vi "Find and Highlight Event Frames.vi"(8 "error in":errorcluster, 10 "References":refnum<vi>[](array[refnum]), 11 "Event Name":string) -> (0 "error out":errorcluster)   [LabVIEW 2019, in "Panther Dashboard.lvlib"]
uses:
  Panther Dashboard.lvlib
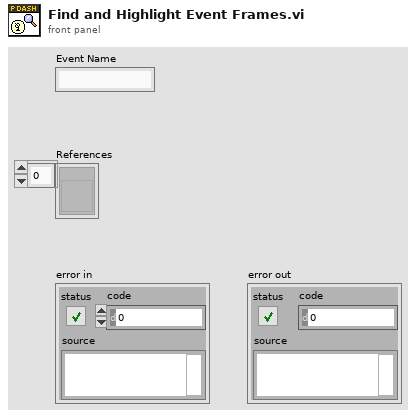
[diagram p1: front panel]
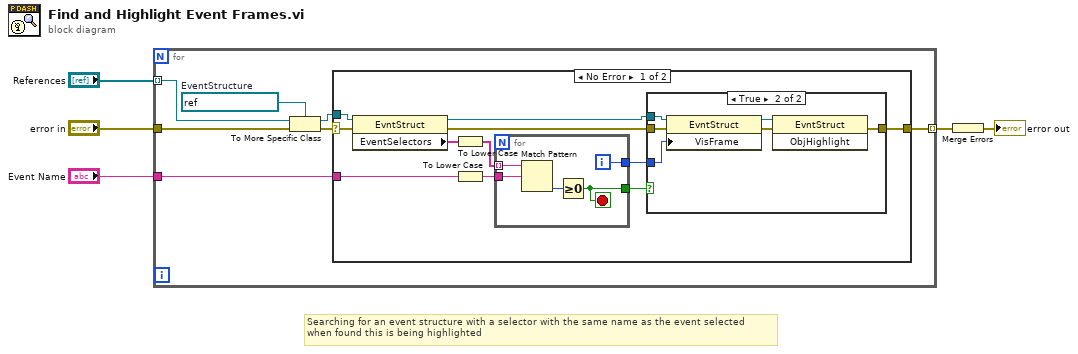
[diagram p0: block diagram]
diagram:
  # "Searching for an event structure with a selector with the same name as the event selected\nwhen found this is being highlighted"
  n1 = for {
    tunnel: "References" -> [w9] mode=indexing
    tunnel: "Event Name" -> [w6]
    tunnel: "error in" -> [w11]
    tunnel: [w10] -> w1 mode=indexing
    w8 = refnum<vi> refnum  # EventStructure
    n2 = To More Specific Class(target class=w8, reference=w9, error in=w11) -> (specific class reference=w7:refnum<vi>, error out=w12:errorcluster)
    n3 = case shown="No Error" w12 {
      selector: w12 -> [w23 _]
      tunnel: w7 -> [w18 _]
      tunnel: w6 -> [w19 _]
      tunnel: [w21 _] -> w10
      frame No Error {
        n4 = property class="EvntStruct"(reference=w18, error in=w23) -> (reference out=w15:refnum<vi>, error out=w22:errorcluster, "EventSelectors"=w20:string[])
        n5 = To Lower Case(string=w20) -> (all lower case string=w14:string[])
        n6 = To Lower Case(string=w19) -> (all lower case string=w13:string)
        n7 = for {
          tunnel: w14 -> [w35] mode=indexing
          tunnel: w13 -> [w34]
          tunnel: [w32] -> w17
          tunnel: [w31] -> w16
          i -> [w32]
          stop <- w31 stop-if-true
          n8 = Match Pattern(string=w35, regular expression=w34) -> (offset past match=w33:i32)  [unwired: 1 in, 3 out]
          n9 = Greater Or Equal To 0?(x=w33) -> (x >= 0?=w31:bool)
        }
        n10 = case shown="True" w16 {
          tunnel: w15 -> [_ w27]
          tunnel: w17 -> [_ w26]
          tunnel: w22 -> [w24 w29]
          tunnel: [w24 w28] -> w21
          frame False {
          }
          frame True {
            n11 = property class="EvntStruct"(reference=w27, error in=w29, "VisFrame"=w26) -> (reference out=w25:refnum<vi>, error out=w30:errorcluster)
            n12 = invoke class="EvntStruct" method="ObjHighlight"(reference=w25, error in=w30) -> (error out=w28:errorcluster)  [unwired: 1 in, 2 out]
          }
        }
      }
      frame Error {
      }
    }
  }
  n13 = Merge Errors(w1) -> (→"error out":errorcluster)
